vi "Core Actor - CLOSE - External Queues_Notifiers.vi"(8 "error in (no error)":errorcluster, 11 "Child_1_Class in":refnum<class "GUI_Class.lvclass">) -> (0 "error out":errorcluster, 3 "Child_1_Class out":refnum<class "GUI_Class.lvclass">)   [LabVIEW 2023, in "GUI_Actor.lvlib" / "GUI_Class.lvclass"]
uses:
  GUI_Class.lvclass
  GUI_Class.lvclass/GUI_Class.ctl
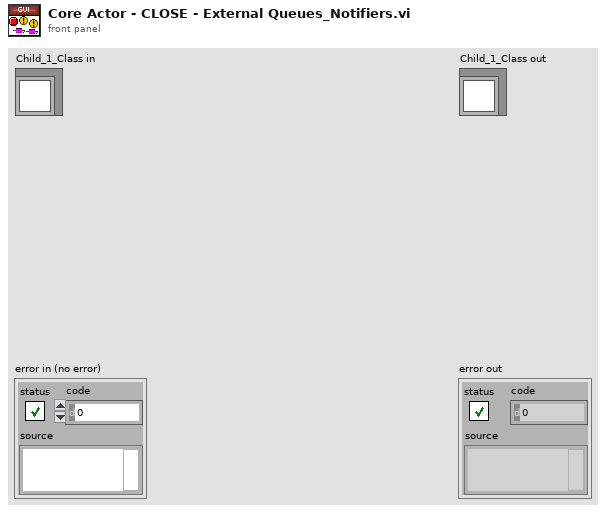
[diagram p1: front panel]
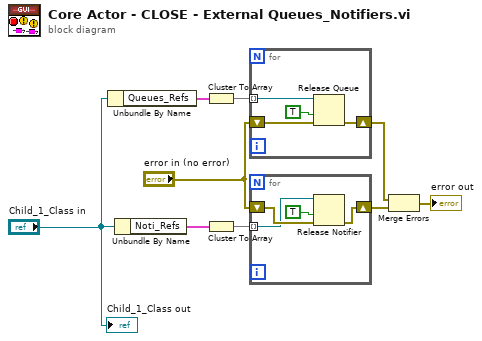
[diagram p0: block diagram]
diagram:
  n1 = Unbundle By Name("Child_1_Class in") -> ("Queues_Refs"=w9:cluster{"TX_QUEUE_REF":refnum<queue>})
  n2 = Unbundle By Name("Child_1_Class in") -> ("Noti_Refs"=w8:cluster{"TX_NOTI_REF":refnum<notifier>})
  n3 = Cluster To Array(cluster=w9) -> (array=w2:refnum<queue>[])
  n4 = Cluster To Array(cluster=w8) -> (array=w1:refnum<notifier>[])
  n5 = for {
    shift-right: [w11] -> w6
    shift-left: "error in (no error)" -> [w12]
    tunnel: w2 -> [w10] mode=indexing
    n6 = Release Queue(queue=w10, force destroy? (F)=TRUE, error in (no error)=w12) -> (error out=w11:errorcluster)  [unwired: 2 out]
  }
  n7 = for {
    shift-right: [w15] -> w5
    shift-left: "error in (no error)" -> [w17]
    tunnel: w1 -> [w14] mode=indexing
    n8 = Release Notifier(notifier=w14, force destroy? (F)=TRUE, error in (no error)=w17) -> (error out=w15:errorcluster)  [unwired: 2 out]
  }
  n9 = Merge Errors(w6, w5) -> (→"error out":errorcluster)
  "Child_1_Class out" <- "Child_1_Class in"
